vi "Verify File.vi"(5 "Label":string, 7 "Options":refnum<class "Options.lvclass">, 8 "error in":errorcluster, 10 "Path to Binary File to Verify":path) -> (0 "error out":errorcluster, 1 "Failure Message":string, 2 "Passed?":bool)   [LabVIEW 2020, in "Approval Tests.lvlib"]
doc: "Takes in a file path. In general compares to approved using the filehash. If it detects a .vi or .ctl file, it uses the built-in comparison function in LabVIEW. In LabVIEW 2020, It is buggy. Apparently some of those bugs have been fixed in newer versions."
uses:
  Approval Tests.lvlib
  Reporter/Reporter.lvclass
  Options/Options.lvclass
  Namer/Namer.lvclass
  File Comparator/File Comparator.lvclass
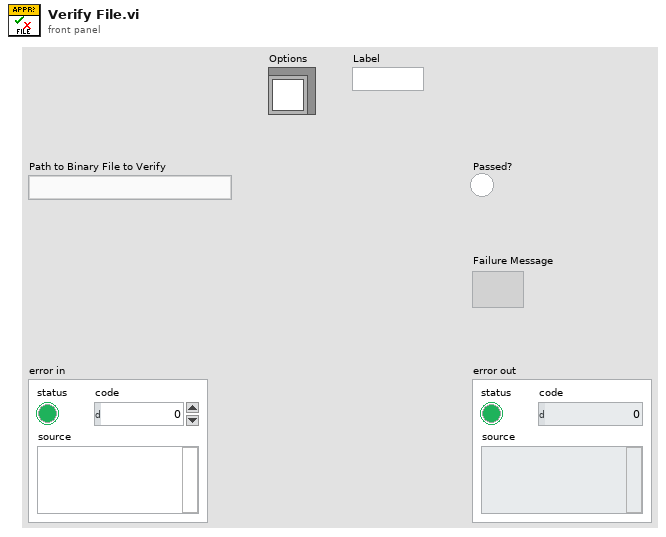
[diagram p1: front panel]
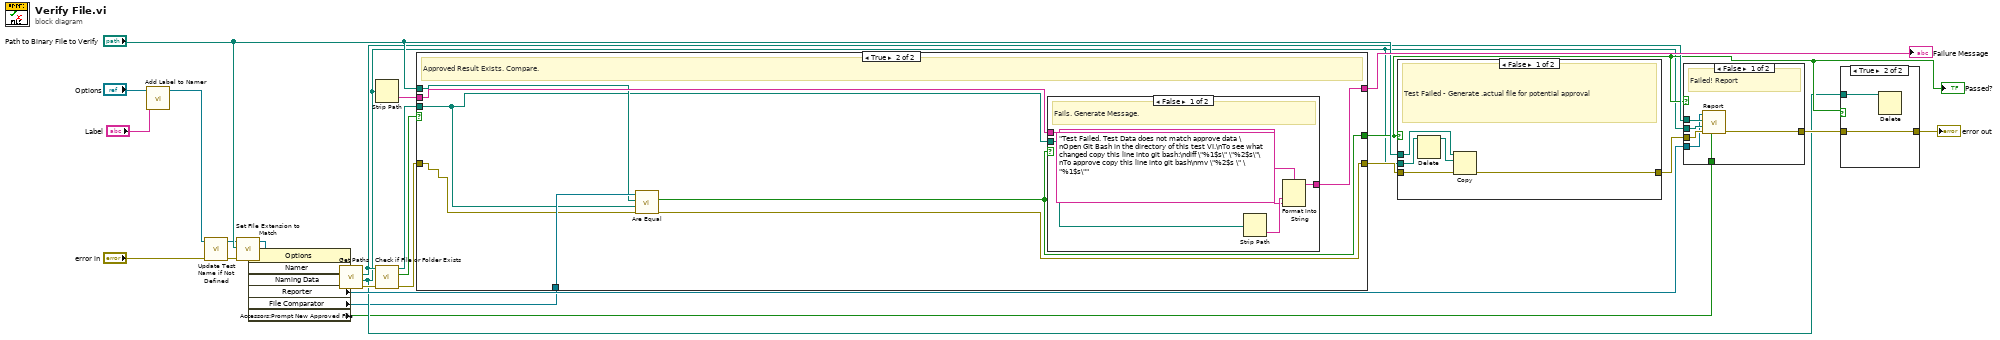
[diagram p0: block diagram]
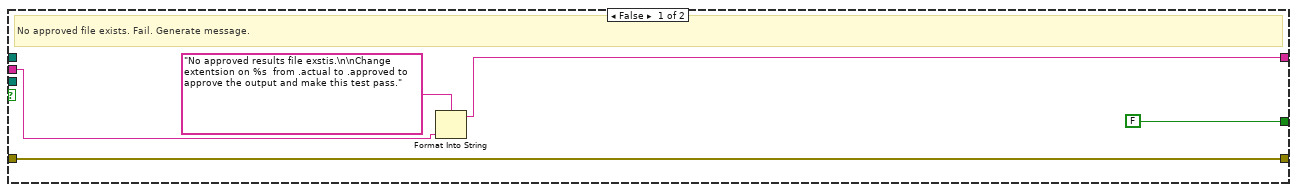
[diagram p5: hidden frame]
diagram:
  n1 = call "Add Label to Namer.vi"("Label"="Label", "Options in"="Options") -> ("Options out"=w4:refnum<class "Options.lvclass">)  [unwired: 9 in]
  n2 = call "Update Test Name if Not Defined.vi"("error in"="error in", "Options in"=w4) -> ("error out"=w23:errorcluster, "Options out"=w10:refnum<class "Options.lvclass">)  [unwired: 8 in]
  n3 = call "Set FIle Extension to Match.vi"("error in"=w23, "Path to Binary File to Verify"="Path to Binary File to Verify", "Options in"=w10) -> ("error out"=w22:errorcluster, "Options out"=w7:refnum<class "Options.lvclass">)  [unwired: 7 in]
  n4 = property class="Options"(reference=w7, error in=w22) -> (error out=w19:errorcluster, "Namer"=w8:refnum<class "Namer.lvclass">, "Naming Data"=w9:refnum<class "Naming Data.lvclass">, "Reporter"=w12:refnum<class "Reporter.lvclass">, "File Comparator"=w2:refnum<class "File Comparator.lvclass">, "Accessors:Prompt New Approved File"=w1:bool)  [unwired: 1 out]
  n5 = call-dynamic "Get Paths.vi"("error in"=w19, "Naming Data"=w9, "Namer in"=w8) -> ("error out"=w24:errorcluster, "Received Path"=w5:path, "Approved Path"=w13:path)  [unwired: 5 in, 1 out]
  n6 = Strip Path(path=w5) -> (name=w15:string)  [unwired: 1 out]
  n7 = call <vilib>:"Check if File or Folder Exists.vi"("error in (no error)"=w24, "path"=w13) -> ("error out"=w28:errorcluster, "file or folder exists?"=w17:bool, "dup path"=w18:path)  [unwired: 7 in]
  n8 = case shown="True" w17 {
    tunnel: [w33 w35] -> w27
    tunnel: w28 -> [w33 w36]
    tunnel: w18 -> [_ w37]
    tunnel: [FALSE ("Passed?") w34] -> w6
    tunnel: [w29 w41] -> w16
    tunnel: w15 -> [w31 w40]
    tunnel: "Path to Binary File to Verify" -> [_ w38]
    tunnel: w2 -> [_ w39]
    frame False {
      # "No approved file exists. Fail. Generate message."
      n9 = Format Into String(format string="No approved results file exstis.\n\nChange extentsion on %s  from .actual to .approved to approve the output and make this test pass.", w31) -> (resulting string=w29:string)  [unwired: 2 in, 1 out]
    }
    frame True {
      # "Approved Result Exists. Compare."
      n10 = call-dynamic "Are Equal.vi"("error in (no error)"=w36, "Recieved File Path"=w37, "Approved File Path"=w38, "File Comparator in"=w39) -> ("error out"=w35:errorcluster, "Are Equal?"=w34:bool)  [unwired: 5 in, 1 out]
      n11 = case shown="False" w34 {
        tunnel: [w46 _] -> w41
        tunnel: w37 -> [w43 _]
        tunnel: w40 -> [w42 _]
        frame False {
          # "Fails. Generate Message."
          n12 = Strip Path(path=w43) -> (name=w44:string)  [unwired: 1 out]
          n13 = Format Into String(format string="Test Failed. Test Data does not match approve data \nOpen Git Bash in the directory of this test VI.\nTo see what changed copy this line into git bash:\ndiff \"%1$s\" \"%2$s\"\nTo approve copy this line into git bash\nmv \"%2$s \" \"%1$s\"", w44, w42) -> (resulting string=w46:string)  [unwired: 2 in, 1 out]
        }
        frame True {
          # "Passes. No Message Needed.."
        }
      }
    }
  }
  "Passed?" <- w6
  "Failure Message" <- w16
  n14 = case shown="False" w6 {
    tunnel: w27 -> [w51 w52]
    tunnel: [w50 w52] -> w26
    tunnel: w5 -> [w49 _]
    tunnel: "Path to Binary File to Verify" -> [w47 _]
    frame False {
      # "Test Failed - Generate .actual file for potential approval"
      n15 = Delete(path (use dialog)=w49) -> (deleted path=w48:path)  [unwired: 4 in, 2 out]
      n16 = Copy(8:w51, 10:w48, 11:w47) -> (0:w50:errorcluster)  [unwired: 2 in, 2 out]
    }
    frame True {
      # "Passed - no need for .actual file"
    }
  }
  n17 = case shown="False" w6 {
    tunnel: w5 -> [w55 _]
    tunnel: w13 -> [w56 _]
    tunnel: w26 -> [w58 w59]
    tunnel: [w57 w59] -> w21
    tunnel: w12 -> [w54 _]
    tunnel: w1 -> [w53 _]
    frame False {
      # "Failed! Report"
      n18 = call "Report.vi"("Prompt to add new approved file to project? (T)"=w53, "error in"=w58, "Received"=w55, "Approved"=w56, "Reporter in"=w54) -> ("error out"=w57:errorcluster)  [unwired: 4 in, 2 out]
    }
    frame True {
      # "Passed - Nothing to Report"
    }
  }
  n19 = case shown="True" w6 {
    tunnel: w21 -> [w60 w62]
    tunnel: [w60 w62] -> w20
    tunnel: w5 -> [_ w61]
    frame False {
    }
    frame True {
      n20 = Delete(path (use dialog)=w61) -> ()  [unwired: 4 in, 3 out]
    }
  }
  "error out" <- w20
